vi "Laurel Read Active Sub1.vi"(0 "TCP Network Connection in":refnum<k5>, 1 "Serial VISA":refnum<visa-resource-name>, 5 "Send Command in":string, 7 "All Items Byte Count (Flow Rate)":i32, 9 "Connection Type":T1, 11 "error in (no error)":errorcluster) -> (3 "VISA resource name 2":refnum<visa-resource-name>, 4 "TCP Network Connection out":refnum<k5>, 6 "return count":u32, 10 "trimmed string":string, 13 "Flow Rate (Item 1)":dbl, 14 "Gallons (Item 2)":dbl, 15 "error out":errorcluster)   [LabVIEW 2019]
uses:
  Type Definitions/Laurel Connection Type.ctl
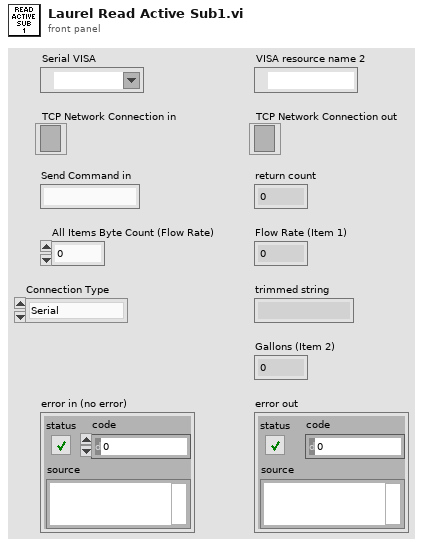
[diagram p1: front panel]
types:
  T1 = typedef "Laurel Connection Type.ctl" = enum16{"Serial", "TCP"}
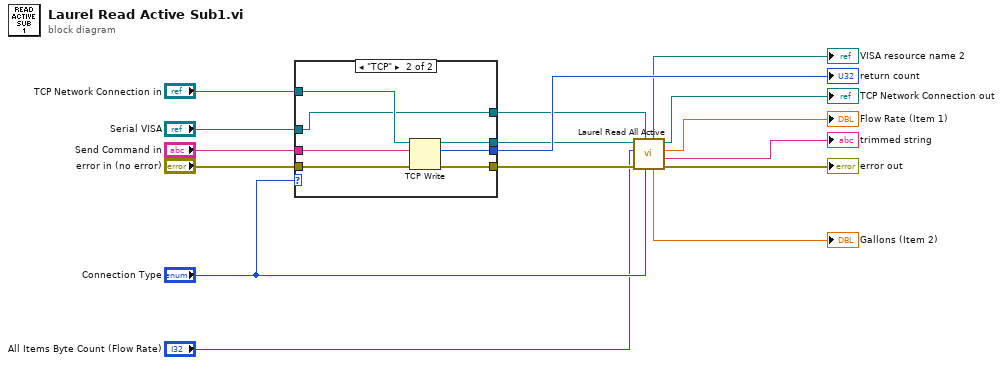
[diagram p0: block diagram]
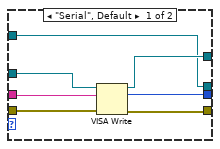
[diagram p2: hidden frame]
diagram:
  n1 = case shown="\"TCP\"" "Connection Type" {
    tunnel: [w19 w30] -> w16
    tunnel: [w22 w29] -> w9
    tunnel: "error in (no error)" -> [w23 w28]
    tunnel: [w17 w27] -> w15
    tunnel: "Send Command in" -> [w21 w26]
    tunnel: [w20 w24] -> w14
    tunnel: "Serial VISA" -> [w18 w24]
    tunnel: "TCP Network Connection in" -> [w17 w25]
    frame "Serial", Default {
      n2 = VISA Write(VISA resource name=w18, write buffer=w21, error in (no error)=w23) -> (VISA resource name out=w20:refnum<visa-resource-name>, return count=w19:u32, error out=w22:errorcluster)
    }
    frame "TCP" {
      n3 = TCP Write(connection ID=w25, data in=w26, error in (no error)=w28) -> (connection ID out=w27:refnum<k5>, bytes written=w30:i32, error out=w29:errorcluster)  [unwired: 1 in]
    }
  }
  "return count" <- w16
  n4 = call "Laurel Read All Active.vi"("Connection Type"="Connection Type", "VISA resource name"=w14, "error in (no error)"=w9, "byte count in"="All Items Byte Count (Flow Rate)", "TCP Network Connection in"=w15) -> ("error out"=→"error out":errorcluster, "trimmed string"=→"trimmed string":string, "Flow Rate (Item 1)"=→"Flow Rate (Item 1)":dbl, "TCP Network Connection out"=→"TCP Network Connection out":refnum<k5>, "Gallons (Item 2)"=→"Gallons (Item 2)":dbl, "VISA resource name 2"=→"VISA resource name 2":refnum<visa-resource-name>)  [unwired: 1 in]
